vi "Main old.vi"(8 "error in (no error)":errorcluster, 11 "Plugin Thread in":refnum<class "Plugin Thread.lvclass">) -> (0 "error out":errorcluster, 3 "Plugin Thread out":refnum<class "Plugin Thread.lvclass">)   [LabVIEW 2017, in "DSF Core.lvlib" / "Plugin Thread.lvclass"]
uses:
  Thread/Plugin/Plugin Thread.lvclass
  Thread Parameters/Thread Parameters.lvclass
  <vilib>/Platform/TimedLoop/XDataNode/wakeup.ctl
  <vilib>/Platform/TimedLoop/XDataNode/XDNodeRunTimeDep.lvlib
  <vilib>/Platform/TimedLoop/XDataNode/nitl_modes.ctl
  <vilib>/Platform/TimedLoop/XDataNode/timing_clust.ctl
  <vilib>/platform/TimedLoop/XDataNode/XDataNode.xnode
panel:
  out "iteration":i32
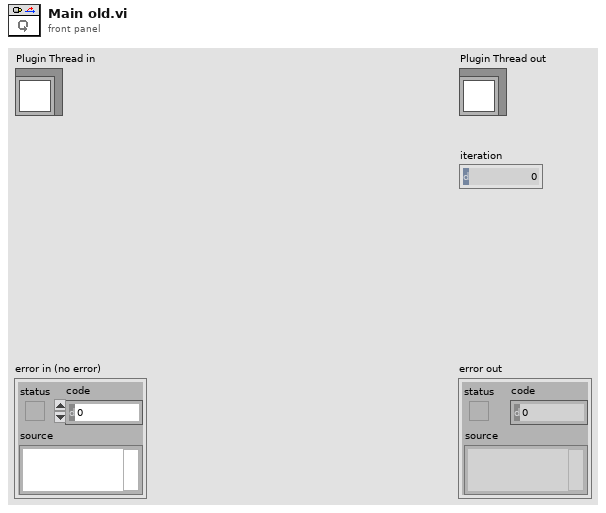
[diagram p1: front panel]
types:
  T1 = typedef "XDNodeRunTimeDep.lvlib/timing_clust.ctl" = cluster{"Expected End [f-1]":u64, "Actual End [f-1]":u64, "Finished Late? [f-1]":bool, "Expected End [i-1]":u64, "Actual End [i-1]":u64, "Finished Late? [i-1]":bool, "Expected Start [i]":u64, "Actual Start [i]":u64, "Expected Start [f]":u64, "Actual Start [f]":u64, "Source Name":string, "Structure Name":string, "Period":i64, "Deadline":i64, "Offset":i64, "Start":i64, "Priority":i32, "Timeout":i32, "Mode":T2, "Wakeup Reason":T3, "Error":errorcluster, "Source Type":string, "Secondary Source Type":string, "Global End Time":u64, "Global Start Time":u64, "Frame Duration":u64, "Iteration Duration":u64, "Assigned CPU":i32, "I/O Scan Engine Mode":u32}
  T2 = typedef "XDNodeRunTimeDep.lvlib/nitl_modes.ctl" = enum32{"No Change", "Process missed periods, maintain original phase", "Discard missed periods, maintain original phase", "Process missed periods, ignore original phase", "Discard missed periods, ignore original phase"}
  T3 = typedef "XDNodeRunTimeDep.lvlib/wakeup.ctl" = enum32{"Normal", "Aborted", "Asynchronous wakeup", "Timing source error", "Timed loop error", "Timeout"}
  T4 = typedef "DSF Core.lvlib/Plugin Interface.lvclass/Command Data.ctl" = cluster{"Command":T5, "Command Parameters":T6}
  T5 = typedef "DSF Core.lvlib/Plugin Interface.lvclass/Command.ctl" = enum8{"Set Base Pointer", "Rx", "Tx", "Shutdown"}
  T6 = typedef "DSF Core.lvlib/Plugin Interface.lvclass/Command Parameters.ctl" = cluster{"arg1":u64, "arg2":u64}
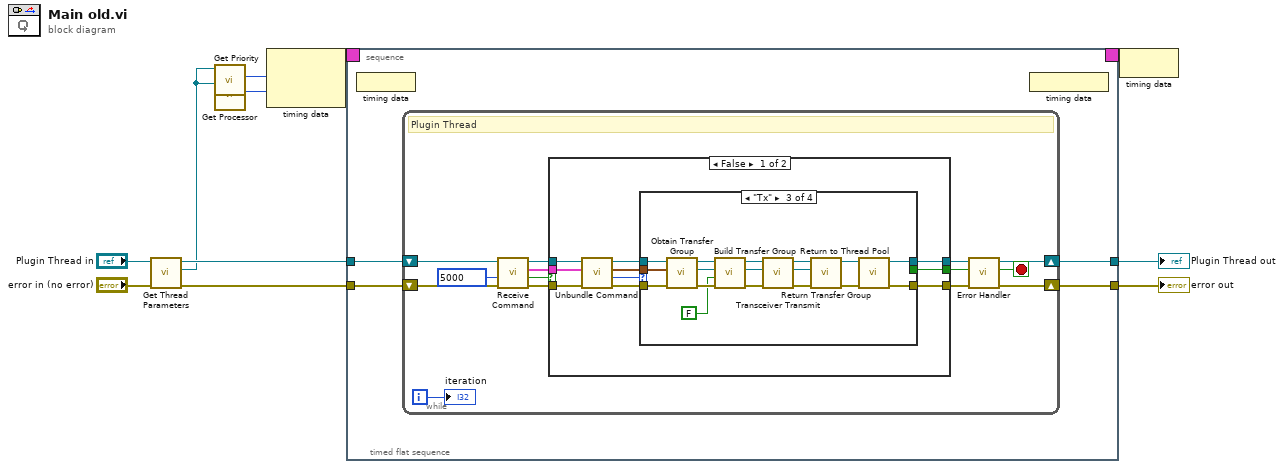
[diagram p0: block diagram]
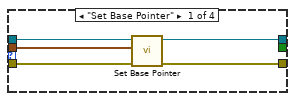
[diagram p2: hidden frame]
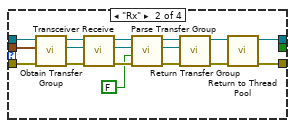
[diagram p3: hidden frame]
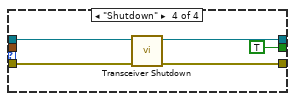
[diagram p4: hidden frame]
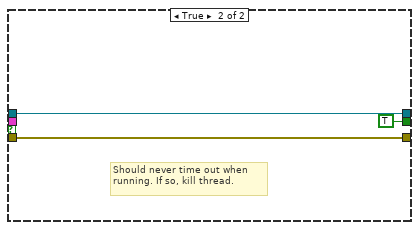
[diagram p5: hidden frame]
diagram:
  n1 = call "Get Thread Parameters.vi"("Transceiver Thread in"="Plugin Thread in") -> ("Thread Parameters"=w3:refnum<class "Thread Parameters.lvclass">, "Transceiver Thread out"=w4:refnum<class "Plugin Thread.lvclass">)  [unwired: 9 in]
  n2 = call "Get Priority.vi"("Thread Parameters in"=w3) -> ("Priority"=w6:i32)  [unwired: 9 in, 1 out]
  n3 = call "Get Processor.vi"("Thread Parameters in"=w3) -> ("Processor"=w5:i32)  [unwired: 9 in, 1 out]
  n4 = node-c288(w6, w5) -> (w10:T1)
  n5 = timed-sequence {
    timing: w10 -> [_]
    timing-out: [_] -> w9
    tunnel: w4 -> [w14]
    tunnel: [w13] -> w8
    tunnel: "error in (no error)" -> [w12]
    tunnel: [w11] -> w1
    n6 = timed-flat-sequence {
      tunnel: w14 -> [w18]
      tunnel: [w17] -> w13
      tunnel: w12 -> [w16]
      tunnel: [w15] -> w11
      n7 = node-c288() -> ()  [unwired: 1 in]
      n8 = while {
        shift-right: [w22] -> w15
        shift-left: w16 -> [w30]
        shift-right: [w23] -> w17
        shift-left: w18 -> [w27]
        i -> [w19]
        stop <- w21 stop-if-true
        # "Plugin Thread"
        n9 = call "Receive Command.vi"("error in (no error)"=w30, "timeout in ms (0)"=5000 ("timeout in ms"), "Plugin Thread in"=w27) -> ("error out"=w26:errorcluster, "timed out?"=w28:bool, "command"=w29:T4, "Plugin Thread out"=w31:refnum<class "Plugin Thread.lvclass">)  [unwired: 5 in]
        n10 = case shown="False" w28 {
          tunnel: w31 -> [w40 w89]
          tunnel: [w42 w89] -> w25
          tunnel: w26 -> [w39 w88]
          tunnel: w29 -> [w38 _]
          tunnel: [w41 w88] -> w24
          tunnel: [w33 TRUE] -> w20
          frame False {
            n11 = call "Unbundle Command.vi"("error in (no error)"=w39, "command"=w38, "Plugin Thread in"=w40) -> ("error out"=w36:errorcluster, "command"=w37:T5, "command parameters"=w34:T6, "Plugin Thread out"=w35:refnum<class "Plugin Thread.lvclass">)  [unwired: 5 in]
            n12 = case shown="\"Tx\"" w37 {
              tunnel: w35 -> [w47 w54 w71 w86]
              tunnel: [w46 w56 w74 w84] -> w42
              tunnel: w36 -> [w43 w49 w70 w85]
              tunnel: w34 -> [w44 w53 w67 _]
              tunnel: [w45 w55 w73 w83] -> w41
              tunnel: [_ _ _ TRUE] -> w33
              frame "Set Base Pointer" {
                n13 = call "Set Base Pointer.vi"("error in (no error)"=w43, "command parameters"=w44, "Plugin Thread in"=w47) -> ("error out"=w45:errorcluster, "Plugin Thread out"=w46:refnum<class "Plugin Thread.lvclass">)  [unwired: 7 in]
              }
              frame "Rx" {
                n14 = call "Obtain Transfer Group.vi"("error in (no error)"=w49, "command parameters"=w53, "Transceiver Thread in"=w54) -> ("error out"=w51:errorcluster, "Transfer Group"=w50:refnum<class "Transfer Group.lvclass">, "Transceiver Thread out"=w52:refnum<class "Plugin Thread.lvclass">)  [unwired: 6 in]
                n15 = call "Transceiver Receive.vi"("error in (no error)"=w51, "Transfer Group in"=w50, "Transceiver Thread in"=w52) -> ("error out"=w63:errorcluster, "Transfer Group out"=w62:refnum<class "Transfer Group.lvclass">, "Transceiver Thread out"=w64:refnum<class "Plugin Thread.lvclass">)  [unwired: 6 in]
                n16 = call "Parse Transfer Group.vi"("error in (no error)"=w63, "inline?"=FALSE, "Transfer Group in"=w62, "Plugin Thread in"=w64) -> ("error out"=w60:errorcluster, "Transfer Group out"=w59:refnum<class "Transfer Group.lvclass">, "Plugin Thread out"=w61:refnum<class "Plugin Thread.lvclass">)  [unwired: 5 in]
                n17 = call "Return Transfer Group.vi"("error in (no error)"=w60, "Transfer Group"=w59, "Transceiver Thread in"=w61) -> ("error out"=w57:errorcluster, "Transceiver Thread out"=w58:refnum<class "Plugin Thread.lvclass">)  [unwired: 7 in]
                n18 = call "Return to Thread Pool.vi"("error in (no error)"=w57, "Plugin Thread in"=w58) -> ("error out"=w55:errorcluster, "Plugin Thread out"=w56:refnum<class "Plugin Thread.lvclass">)  [unwired: 8 in]
              }
              frame "Tx" {
                n19 = call "Obtain Transfer Group.vi"("error in (no error)"=w70, "command parameters"=w67, "Transceiver Thread in"=w71) -> ("error out"=w68:errorcluster, "Transfer Group"=w66:refnum<class "Transfer Group.lvclass">, "Transceiver Thread out"=w69:refnum<class "Plugin Thread.lvclass">)  [unwired: 6 in]
                n20 = call "Build Transfer Group.vi"("error in (no error)"=w68, "inline?"=FALSE, "Transfer Group in"=w66, "Plugin Thread in"=w69) -> ("error out"=w80:errorcluster, "Transfer Group out"=w72:refnum<class "Transfer Group.lvclass">, "Plugin Thread out"=w81:refnum<class "Plugin Thread.lvclass">)  [unwired: 5 in]
                n21 = call "Transceiver Transmit.vi"("error in (no error)"=w80, "Transfer Group in"=w72, "Transceiver Thread in"=w81) -> ("error out"=w78:errorcluster, "Transfer Group out"=w77:refnum<class "Transfer Group.lvclass">, "Transceiver Thread out"=w79:refnum<class "Plugin Thread.lvclass">)  [unwired: 6 in]
                n22 = call "Return Transfer Group.vi"("error in (no error)"=w78, "Transfer Group"=w77, "Transceiver Thread in"=w79) -> ("error out"=w75:errorcluster, "Transceiver Thread out"=w76:refnum<class "Plugin Thread.lvclass">)  [unwired: 7 in]
                n23 = call "Return to Thread Pool.vi"("error in (no error)"=w75, "Plugin Thread in"=w76) -> ("error out"=w73:errorcluster, "Plugin Thread out"=w74:refnum<class "Plugin Thread.lvclass">)  [unwired: 8 in]
              }
              frame "Shutdown" {
                n24 = call "Transceiver Shutdown.vi"("error in (no error)"=w85, "Transceiver Thread in"=w86) -> ("error out"=w83:errorcluster, "Transceiver Thread out"=w84:refnum<class "Plugin Thread.lvclass">)  [unwired: 8 in]
              }
            }
          }
          frame True {
            # "Should never time out when running. If so, kill thread."
          }
        }
        n25 = call "Error Handler.vi"("error in (no error)"=w24, "stop"=w20, "Plugin Thread in"=w25) -> ("error out"=w22:errorcluster, "stop"=w21:bool, "Plugin Thread out"=w23:refnum<class "Plugin Thread.lvclass">)  [unwired: 6 in]
        "iteration" <- w19
      }
      n26 = node-c288() -> ()  [unwired: 1 out]
    }
  }
  "error out" <- w1
  "Plugin Thread out" <- w8
  n27 = node-c288(w9) -> ()
